vi "Channel Basics Lesson 1.vi"() -> ()   [LabVIEW 2023]
doc: "This VI demonstrates basic use a Stream channel, the first channel kind that users will see in this example."
uses:
  <extravilib>/ChannelInstances/Stream-i32/Read With Abort.vi
  <extravilib>/ChannelInstances/Stream-i32/Write With Abort.vi
  <extravilib>/ChannelInstances/Stream-i32/EndpointRead.vi
  <extravilib>/ChannelInstances/Stream-i32/Endpoint.vi
  <extravilib>/ChannelInstances/Stream-i32/Instantiate.vi
  <extravilib>/ChannelInstances/Stream-i32/)Channel.vi
  <resource>/ChannelSupport/_ChannelSupport/WaitIfNeeded.vi
  <extravilib>/ChannelInstances/Stream-i32.lvlib
panel:
  in  "Stop Writer B":bool
  out "Writer B":i32(graph)
  in  "Stop Reader B":bool
  out "Reader B":i32(graph)
  in  "Stop Reader A":bool
  out "Reader A":i32(graph)
  in  "Stop Writer A":bool
  out "Writer A":i32(graph)
  # "Overview: This VI demonstrates how to use channel wires. \n\nChannels are not like normal dataflow wires. When a dataflow wire connects two nodes, it means that the downstream node must wait for data from the upstream node before it can execute. Channels are asynchronous connections. They allow data to be connected between two sections of code running in parallel. \n\nThe channel wire expresses a protocol for transmitting data between the two sections of code, the same way that a queue or a shared variable does, but channels do so with a more direct graphical notation. The advantage is that the channels often require fewer nodes to set up and may combine several signals together in one package to handle cases where the receiver needs to talk back to the sender, without introducing some of the complex wiring often required by traditional methods. Channel wires can even form cycles among nodes, whereas dataflow wires would break.\n\nInstructions:\n1. Open the block diagram. Review the lessons presented there.\n2. Run the VI to see that the behavior of the queue implementation (above) is the same as the channel implementation (below).\n3. To stop the loops, you must stop the Reader loops before the Writer loops or this example will hang, by design. If you forget, use the Abort button to stop the example. Lesson 2 addresses this issue."
  # "Remember to stop readers before writers!"
  # "Remember to stop readers before writers!"
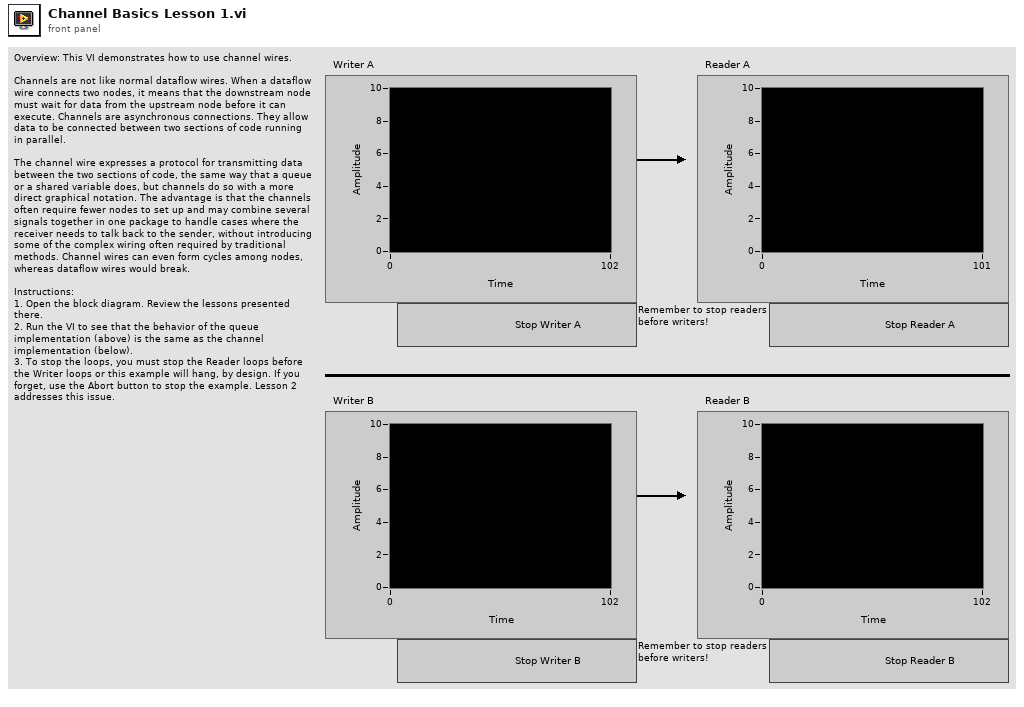
[diagram p1: front panel]
types:
  T1 = typedef "Stream-i32.lvlib/)Channel.ctl" = refnum<queue>
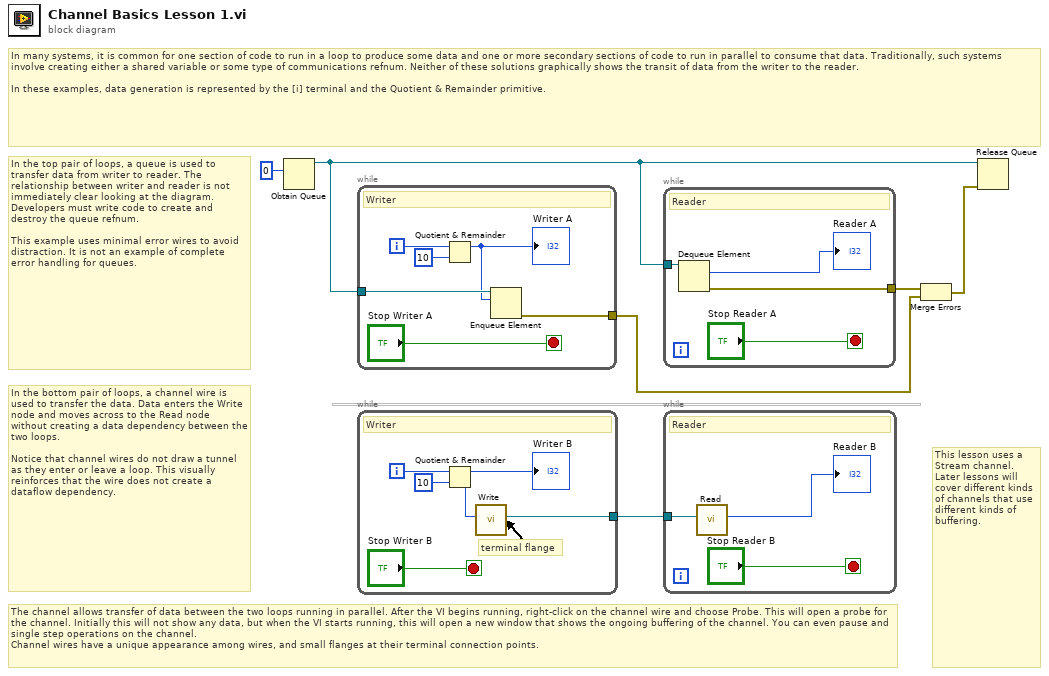
[diagram p0: block diagram]
diagram:
  # "This lesson uses a Stream channel. Later lessons will cover different kinds of channels that use different kinds of buffering."
  # "The channel allows transfer of data between the two loops running in parallel. After the VI begins running, right-click on the channel wire and choose Probe. This will open a probe for the channel. Initially this will not show any data, but when the VI starts running, this will open a new window that shows the ongoing buffering of the channel. You can even pause and single step operations on the channel.\nChannel wires have a unique appearance among wires, and small flanges at their terminal connection points."
  # "In the bottom pair of loops, a channel wire is used to transfer the data. Data enters the Write node and moves across to the Read node without creating a data dependency between the two loops.\n\nNotice that channel wires do not draw a tunnel as they enter or leave a loop. This visually reinforces that the wire does not create a dataflow dependency."
  # "In the top pair of loops, a queue is used to transfer data from writer to reader. The relationship between writer and reader is not immediately clear looking at the diagram. Developers must write code to create and destroy the queue refnum.\n\nThis example uses minimal error wires to avoid distraction. It is not an example of complete error handling for queues."
  # "In many systems, it is common for one section of code to run in a loop to produce some data and one or more secondary sections of code to run in parallel to consume that data. Traditionally, such systems involve creating either a shared variable or some type of communications refnum. Neither of these solutions graphically shows the transit of data from the writer to the reader.\n\nIn these examples, data generation is represented by the [i] terminal and the Quotient & Remainder primitive."
  n1 = Obtain Queue(element data type=0 ("y")) -> (queue out=w5:refnum<queue>)  [unwired: 4 in, 2 out]
  n2 = while {
    tunnel: w5 -> [w9]
    tunnel: [w7] -> w3
    i -> [w11]
    stop <- "Stop Writer A" stop-if-true
    # "Writer"
    n3 = Quotient & Remainder(x=w11, y=10) -> (x-y*floor(x/y)=w8:i32)  [unwired: 1 out]
    "Writer A" <- w8
    n4 = Enqueue Element(queue=w9, element=w8) -> (error out=w7:errorcluster)  [unwired: 2 in, 2 out]
  }
  n5 = while {
    tunnel: [w13] -> w1
    i -> [w16]
    stop <- "Stop Writer B" stop-if-true
    # "terminal flange"
    # "Writer"
    n6 = Quotient & Remainder(x=w16, y=10) -> (x-y*floor(x/y)=w14:i32)  [unwired: 1 out]
    "Writer B" <- w14
    n7 = call <extravilib>:"Write.vi"("element"=w14) -> ("channel"=w13:T1)  [unwired: 8 in, 2 out]
  }
  n8 = while {
    tunnel: w5 -> [w20]
    tunnel: [w18] -> w4
    stop <- "Stop Reader A" stop-if-true
    # "Reader"
    n9 = Dequeue Element(queue=w20) -> (element=→"Reader A":i32, error out=w18:errorcluster)  [unwired: 2 in, 2 out]
  }
  n10 = while {
    tunnel: w1 -> [w23]
    stop <- "Stop Reader B" stop-if-true
    # "Reader"
    n11 = call <extravilib>:"Read.vi"("channel"=w23) -> ("element"=→"Reader B":i32)  [unwired: 6 in, 4 out]
  }
  n12 = Merge Errors(w4, w3) -> (w2:errorcluster)
  n13 = Release Queue(queue=w5, error in (no error)=w2) -> ()  [unwired: 1 in, 3 out]
